vi "New Line to File.vi"(10 "Output File":path, 11 "Text to add":string) -> ()   [LabVIEW 2010]
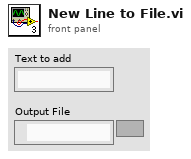
[diagram p1: front panel]
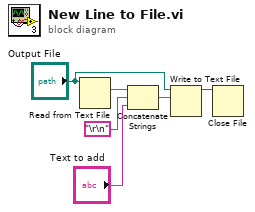
[diagram p0: block diagram]
diagram:
  n1 = Read from Text File(file (use dialog)="Output File") -> (text=w3:string)  [unwired: 3 in, 3 out]
  n2 = Concatenate Strings(w3, "\r\n", "Text to add") -> (w4:string)
  n3 = Write to Text File(file (use dialog)="Output File", text=w4) -> (refnum out=w2:refnum<file>)  [unwired: 2 in, 2 out]
  n4 = Close File(refnum=w2) -> ()  [unwired: 1 in, 2 out]
